vi "Manual Override.vi"(6 "Target Auto Angle":T1 scale format="%.3f", 7 "Overide":T2 {"Target Auto Angle" scale format="%.3f"; "Direction"."Rotate(Yaw) CCW 1 CW -1" scale=1.0..-1.0; "Direction"."Traverse"."Angle" scale format="%.3f"; "Direction"."Traverse"."Velocity" scale=-1.0..1.0 scale format="%.1f"}, 8 "CMD Override":T8(ring), 9 "Override":bool, 11 "Auto CMD":T2 {"Target Auto Angle" scale format="%.3f"; "Direction"."Rotate(Yaw) CCW 1 CW -1" scale=1.0..-1.0; "Direction"."Traverse"."Angle" scale format="%.3f"; "Direction"."Traverse"."Velocity" scale=-1.0..1.0 scale format="%.1f"}) -> (3 "OverRide Command Out":T2 {"Target Auto Angle" scale format="%.3f"; "Direction"."Rotate(Yaw) CCW 1 CW -1" scale=1.0..-1.0; "Direction"."Traverse"."Angle" scale format="%.3f"; "Direction"."Traverse"."Velocity" scale=-1.0..1.0 scale format="%.1f"})   [LabVIEW 2023, in "2024 AdvSwerve_ACT.lvlib"]
uses:
  2024 AdvSwerve_ACT.lvlib
  ENUM_CMD_Mode Select.ctl
  Shared Code/TypeDefs/Level_Velocity plus-minus 1.ctl
  Shared Code/TypeDefs/Dial_Compase heading unit circle CCW positive.ctl
  Shared Code/TypeDefs/Cluster_Module Velocity-Direction-Rotations.ctl
  Shared Code/TypeDefs/Cluster_CMD_Direction Data.ctl
  Cluster_CMD_ACT_Data.ctl
  Shared Code/TypeDefs/Cluster_X-Y.ctl
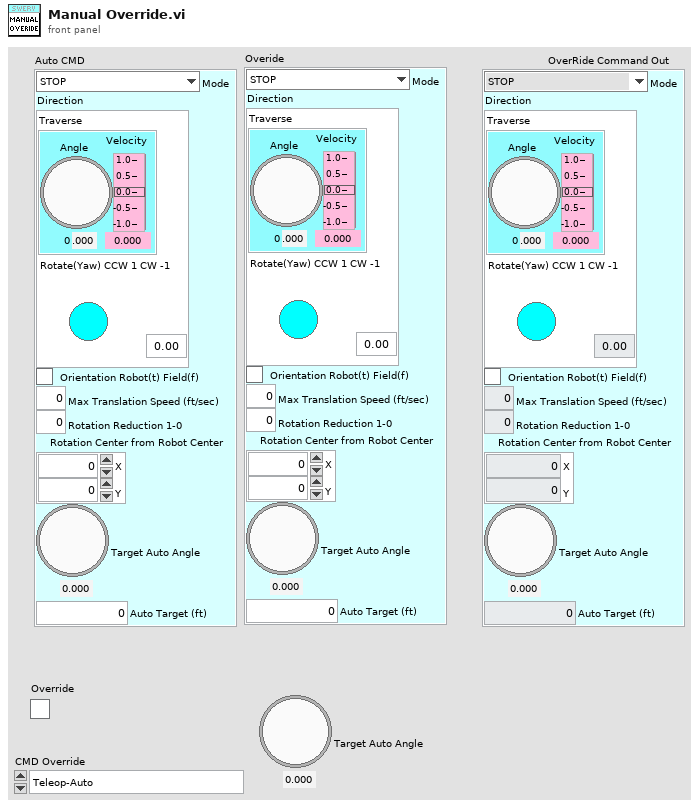
[diagram p1: front panel]
types:
  T1 = typedef "Dial_Compase heading unit circle CCW positive.ctl" = dbl
  T2 = typedef "2024 AdvSwerve_ACT.lvlib/Cluster_CMD_ACT_Data.ctl" = cluster{"Mode":T3, "Direction":T4, "Orientation Robot(t) Field(f)":bool, "Max Translation Speed (ft/sec)":dbl, "Rotation Reduction 1-0":dbl, "Rotation Center from Robot Center":T7, "Target Auto Angle":T1, "Auto Target (ft)":dbl}
  T3 = typedef "2024 AdvSwerve_ACT.lvlib/ENUM_CMD_Mode Select.ctl" = enum16{"STOP", "Move", "Turret Manual", "Trans Manual Angle Auto", "Turret Auto Angle"}
  T4 = typedef "Cluster_CMD_Direction Data.ctl" = cluster{"Traverse":T5, "Rotate(Yaw) CCW 1 CW -1":dbl}
  T5 = typedef "Cluster_Module Velocity-Direction-Rotations.ctl" = cluster{"Velocity":T6, "Angle":T1, "Rotations Count":dbl}
  T6 = typedef "Level_Velocity plus-minus 1.ctl" = dbl
  T7 = typedef "Cluster_X-Y.ctl" = cluster{"X":dbl, "Y":dbl}
  T8 = enum32{"Teleop-Auto", "OverideAll", "AutoRotate", "STOP"}
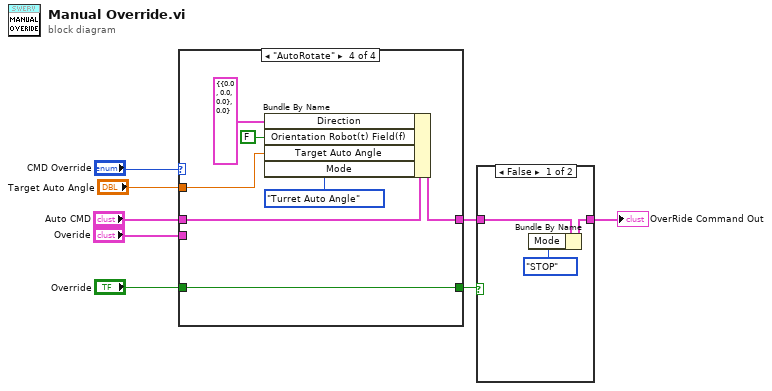
[diagram p0: block diagram]
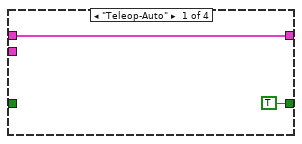
[diagram p3: hidden frame]
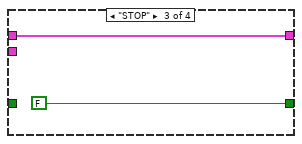
[diagram p5: hidden frame]
diagram:
  n1 = case shown="\"AutoRotate\"" "CMD Override" {
    tunnel: [w10 w12 w14 w18] -> w4
    tunnel: "Auto CMD" -> [w10 _ w14 w19]
    tunnel: "Overide" -> [_ w12 _ _]
    tunnel: "Target Auto Angle" -> [_ _ _ w17]
    tunnel: "Override" -> [_ w11 _ w15]
    tunnel: [TRUE ("Override") w11 FALSE ("Override") w15] -> w1
    frame "Teleop-Auto" {
    }
    frame "OverideAll" {
    }
    frame "STOP" {
    }
    frame "AutoRotate" {
      n2 = Bundle By Name(cluster=w19, "Direction"=T4 {"Traverse"={"Velocity"=0.0, "Angle"=0.0, "Rotations Count"=0.0}, "Rotate(Yaw) CCW 1 CW -1"=0.0}, "Orientation Robot(t) Field(f)"=FALSE, "Target Auto Angle"=w17, "Mode"=ENUM_CMD_Mode_Select."Turret Auto Angle" ("t")) -> (w18:T2)
    }
  }
  n3 = case shown="False" w1 {
    tunnel: w4 -> [w24 w25]
    tunnel: [w23 w25] -> w3
    frame False {
      n4 = Bundle By Name(cluster=w24, "Mode"=ENUM_CMD_Mode_Select."STOP") -> (w23:T2)
    }
    frame True {
    }
  }
  "OverRide Command Out" <- w3
